vi "smaller_greater.vi"(2 "input 2":dbl, 3 "input 1":dbl) -> (0 "greater":dbl, 1 "smaller":dbl)   [LabVIEW 2015]
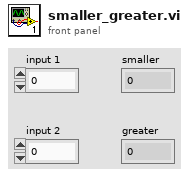
[diagram p1: front panel]
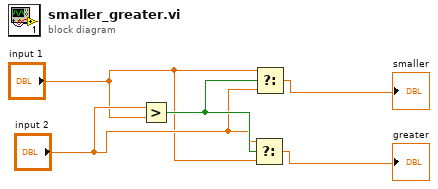
[diagram p0: block diagram]
diagram:
  n1 = Greater?(x="input 2", y="input 1") -> (0:w5:bool)
  n2 = Select(t="input 2", s=w5, f="input 1") -> (s? t:f=→"greater":dbl)
  n3 = Select(t="input 1", s=w5, f="input 2") -> (s? t:f=→"smaller":dbl)
